vi "Search for Model.vi"(0 "Barcode Scan":string, 11 "error in (no error)":errorcluster) -> (4 "Model Number":string, 6 "Model Found?":bool, 8 "Report Text":string, 15 "error out":errorcluster)   [LabVIEW 2016]
doc: "This VI searches the Model Config file for the model number read by the barcode scanner."
uses:
  <vilib>/Utility/error.llb/Error Cluster From Error Code.vi
  <vilib>/ErrorRing/Error Ring.xnode
  <vilib>/Utility/config.llb/NI_LVConfig.lvlib
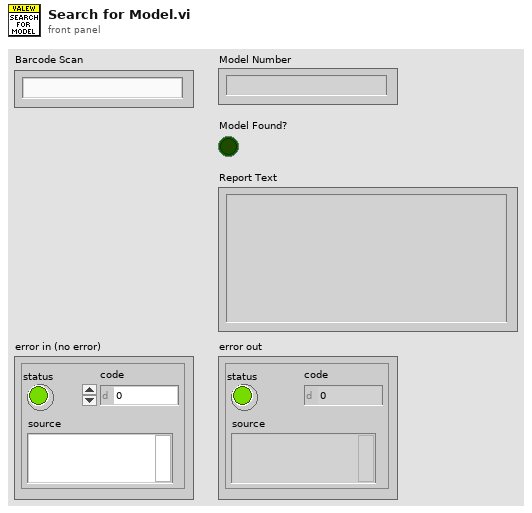
[diagram p1: front panel]
types:
  T1 = typedef "NI_LVConfig.lvlib/Config Data RefNum.ctl" = refnum<k1>
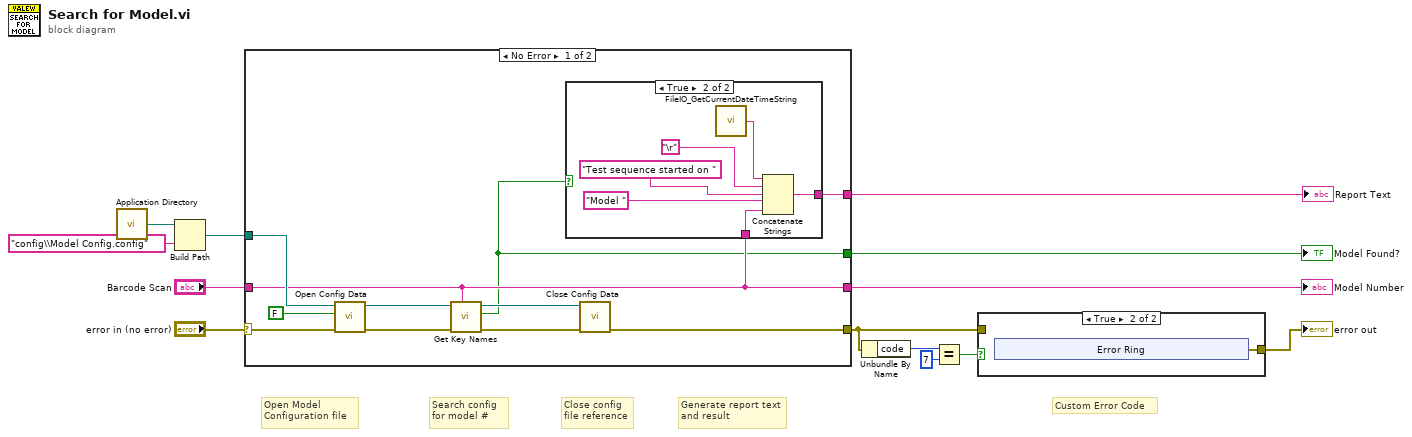
[diagram p0: block diagram]
diagram:
  # "Custom Error Code"
  # "Generate report text\nand result"
  # "Close config\nfile reference"
  # "Search config \nfor model #"
  # "Open Model \nConfiguration file"
  n1 = call <vilib>:"Application Directory.vi"() -> ("Application Directory"=w11:path)
  n2 = Build Path(base path=w11, name or relative path="config\\Model Config.config") -> (appended path=w9:path)
  n3 = case shown="No Error" "error in (no error)" {
    selector: "error in (no error)" -> [w17 w31]
    tunnel: "Barcode Scan" -> [w16 _]
    tunnel: [w21 w31] -> w1
    tunnel: [w14 _] -> w10
    tunnel: w9 -> [w18 _]
    tunnel: [w16 _] -> w7
    tunnel: [w15 _] -> w6
    frame No Error {
      n4 = call <vilib>:"Open Config Data.vi"("error in (no error)"=w17, "create file if necessary (T)"=FALSE, "configuration file path"=w18) -> ("error out"=w23:errorcluster, "refnum"=w24:T1)  [unwired: 6 in, 1 out]
      n5 = call <vilib>:"Get Key Names.vi"("section"=w16, "error in (no error)"=w23, "refnum"=w24) -> ("error out"=w19:errorcluster, "section exists?"=w14:bool, "refnum out"=w20:T1)  [unwired: 5 in, 1 out]
      n6 = case shown="True" w14 {
        tunnel: w16 -> [_ w29]
        tunnel: [_ w27] -> w15
        frame False {
        }
        frame True {
          n7 = call "FileIO_GetCurrentDateTimeString.vi"() -> ("Date/Time String"=w26:string)  [unwired: 14 in, 1 out]
          n8 = Concatenate Strings(w26, "\r", "Test sequence started on ", "Model ", w29) -> (w27:string)
        }
      }
      n9 = call <vilib>:"Close Config Data.vi"("error in (no error)"=w19, "refnum"=w20) -> ("error out"=w21:errorcluster)  [unwired: 8 in, 1 out]
    }
    frame Error {
    }
  }
  "Model Found?" <- w10
  "Model Number" <- w7
  "Report Text" <- w6
  n10 = Unbundle By Name(w1) -> ("code"=w5:i32)
  n11 = Equal?(x=w5, y=7) -> (x = y?=w3:bool)
  n12 = case shown="True" w3 {
    tunnel: [w32 w33] -> w2
    tunnel: w1 -> [w32 _]
    frame False {
    }
    frame True {
      n13 = xnode "Error Ring"() -> ("error out"=w33:errorcluster)
    }
  }
  "error out" <- w2
